vi "SendEmail.vi"(0 "File path":path[](array[path]), 1 "Body":string, 2 "Subject":string, 3 "Receive Adress":string[](array[string])) -> ()   [LabVIEW 2022 SP3]
uses:
  <vilib>/smtpClient/Set Message Text.vi
  <vilib>/smtpClient/LabVIEWSMTPClient.lvlib
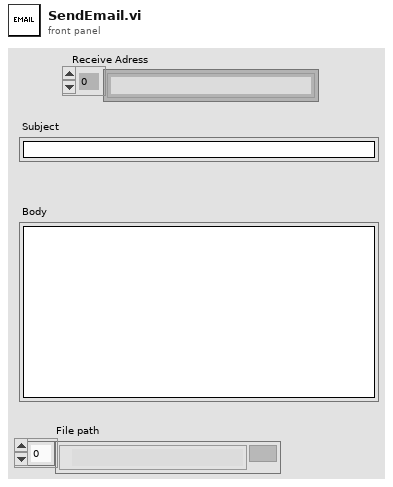
[diagram p1: front panel]
types:
  T1 = typedef "LabVIEWSMTPClient.lvlib/SmtpClientHandle.ctl" = refnum<k1>
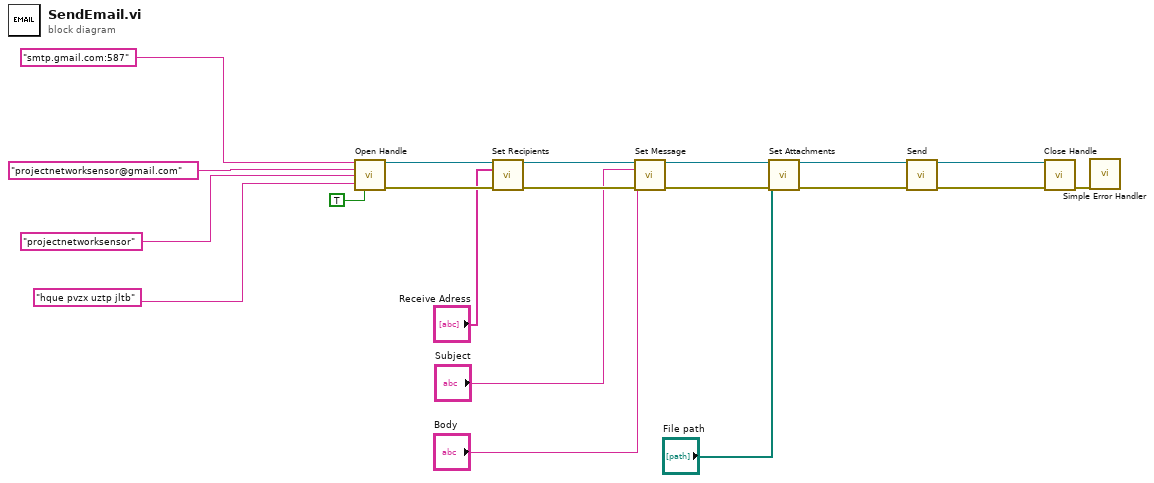
[diagram p0: block diagram]
diagram:
  n1 = call <vilib>:"Open Handle.vi"("server address"="smtp.gmail.com:587", "from"="projectnetworksensor@gmail.com", "username"="projectnetworksensor", "password"="hque pvzx uztp jltb", "use TLS (false)"=TRUE) -> ("handle out"=w20:T1, "error out"=w19:errorcluster)  [unwired: 9 in]
  n2 = call <vilib>:"Set Recipients.vi"("handle in"=w20, "to"="Receive Adress", "error in (no error)"=w19) -> ("handle out"=w18:T1, "error out"=w17:errorcluster)  [unwired: 11 in]
  n3 = call-poly <vilib>:"Set Message.vi"("handle in"=w18, "subject"="Subject", "plain text message"="Body", "error in (no error)"=w17) -> ("handle out"=w16:T1, "error out"=w15:errorcluster)  [unwired: 10 in]
  n4 = call <vilib>:"Set Attachments.vi"("handle in"=w16, "attachments"="File path", "error in (no error)"=w15) -> ("handle out"=w14:T1, "error out"=w13:errorcluster)  [unwired: 11 in]
  n5 = call <vilib>:"Send.vi"("handle in"=w14, "error in (no error)"=w13) -> ("handle out"=w12:T1, "error out"=w11:errorcluster)  [unwired: 11 in, 1 out]
  n6 = call <vilib>:"Close Handle.vi"("handle in"=w12, "error in (no error)"=w11) -> ("error out"=w5:errorcluster)  [unwired: 12 in, 1 out]
  n7 = call <vilib>:"Simple Error Handler.vi"("error in (no error)"=w5) -> ()  [unwired: 4 in, 5 out]
